vi "Close.vi"(8 "error in":errorcluster, 11 "Nominal Value in":refnum<class "Nominal Value.lvclass">) -> (0 "error out":errorcluster, 3 "Nominal Value out":refnum<class "Nominal Value.lvclass">)   [LabVIEW 2023, in "Nominal Value.lvclass"]
uses:
  Nominal Value.lvclass
  Nominal Value.lvclass/Nominal Value.ctl
  <vilib>/ADAS Replay HIL/AdasHilServices/AdasHilServices Fill In Error Info Ex.vi
  <vilib>/ADAS Replay HIL/AdasHilServices/AdasHilChannelServices.lvlib
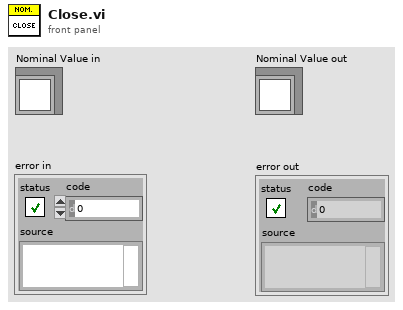
[diagram p1: front panel]
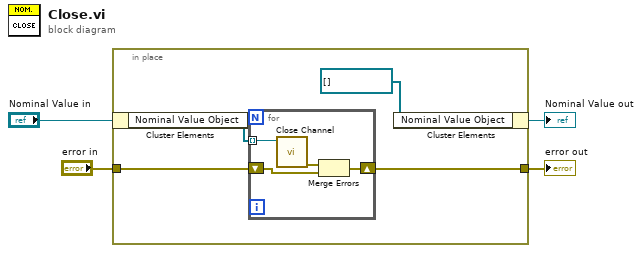
[diagram p0: block diagram]
diagram:
  n1 = in-place {
    in-place-border: [w8] -> w4
    in-place-border: "error in" -> [w5]
    n2 = in-place-cluster #1("Nominal Value in") -> ("Nominal Value Object"=w7:refnum<k21>[])
    n3 = for {
      tunnel: w7 -> [w12] mode=indexing
      shift-right: [w9] -> w8
      shift-left: w5 -> [w10]
      n4 = call <vilib>:"Close Channel.vi"("ADAS HIL Channel"=w12) -> ("error out"=w11:errorcluster)  [unwired: 10 in]
      n5 = Merge Errors(w11, w10) -> (w9:errorcluster)
    }
    n6 = in-place-cluster #1("Nominal Value Object"=refnum<k21>[] [] ("Actual Value Object")) -> (→"Nominal Value out":refnum<class "Nominal Value.lvclass">)
  }
  "error out" <- w4
